vi "KML-wpDataParseOut.vi"(7 "wp data in":string) -> (0 "alt":string, 2 "lat":string, 3 "lon":string, 5 "wp#":string)   [LabVIEW 8.6]
uses:
  <vilib>/Utility/error.llb/whitespace.ctl
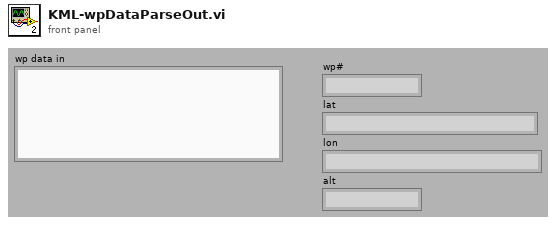
[diagram p1: front panel]
types:
  T1 = typedef "whitespace.ctl" = u16
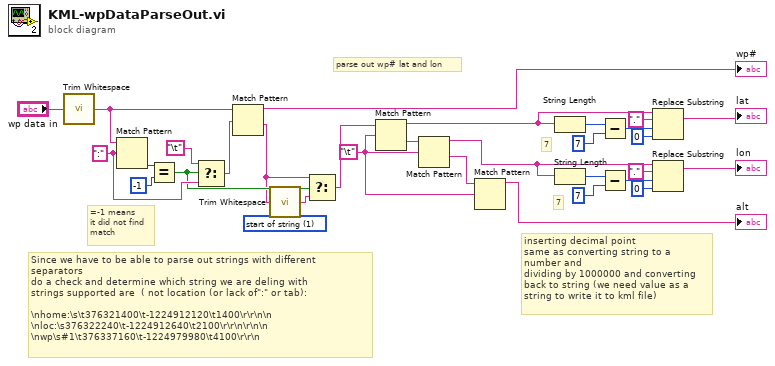
[diagram p0: block diagram]
diagram:
  w3 = T1 1 items=["both", "start of string", "end of string"] ("location (both)")
  w7 = ":" ("regular expression")
  w29 = "\t"
  # "7"
  # "7"
  # "Since we have to be able to parse out strings with different separators\ndo a check and determine which string we are deling with\nstrings supported are  ( not location (or lack of\":\" or tab):\n\n\\nhome:\\s\\t376321400\\t-1224912120\\t1400\\r\\r\\n\\n\n\\nloc:\\s376322240\\t-1224912640\\t2100\\r\\r\\n\\r\\n\\n\n\\nwp\\s#1\\t376337160\\t-1224979980\\t4100\\r\\r\\n"
  # "=-1 means\nit did not find\nmatch"
  # "inserting decimal point\nsame as converting string to a number and\ndividing by 1000000 and converting back to string (we need value as a string to write it to kml file)"
  # "parse out wp# lat and lon"
  n1 = call <vilib>:"Trim Whitespace.vi"("string"="wp data in") -> ("trimmed string"=w11:string)  [unwired: 1 in]
  n2 = Match Pattern(string=w11, regular expression=w7) -> (offset past match=w10:i32)  [unwired: 1 in, 3 out]
  n3 = Equal?(x=w10, y=-1) -> (x = y?=w5:bool)
  n4 = Select(t="\t", s=w5, f=w7) -> (s? t:f=w6:string)
  n5 = Match Pattern(string=w11, regular expression=w6) -> (before substring=→"wp#":string, after substring=w2:string)  [unwired: 1 in, 2 out]
  n6 = call <vilib>:"Trim Whitespace.vi"("string"=w2, "location (both)"=w3) -> ("trimmed string"=w1:string)
  n7 = Select(t=w2, s=w5, f=w1) -> (s? t:f=w4:string)
  n8 = Match Pattern(string=w4, regular expression=w29) -> (before substring=w18:string, after substring=w13:string)  [unwired: 1 in, 2 out]
  n9 = Match Pattern(string=w13, regular expression=w29) -> (before substring=w28:string, after substring=w31:string)  [unwired: 1 in, 2 out]
  n10 = Match Pattern(string=w31, regular expression=w29) -> (before substring=→"alt":string)  [unwired: 1 in, 3 out]
  n11 = String Length(string=w18) -> (length=w14:i32)
  n12 = String Length(string=w28) -> (length=w20:i32)
  n13 = Subtract(x=w14, y=7) -> (x-y=w16:i32)
  n14 = Subtract(x=w20, y=7) -> (x-y=w22:i32)
  n15 = Replace Substring(2:0 ("length (len. of substring)"), 3:w16, 4:"." ("substring (\"\")"), 5:w18) -> (1:→"lat":string)  [unwired: 1 out]
  n16 = Replace Substring(2:0 ("length (len. of substring)"), 3:w22, 4:"." ("substring (\"\")"), 5:w28) -> (1:→"lon":string)  [unwired: 1 out]
